vi "Send Core.vi"(6 "Severity Code (info)":T1=enum."info", 8 "Error In":errorcluster, 9 "Message Content":string, 10 "Message Tag":string, 11 "CS++Syslog in":refnum<class "CS++Syslog.lvclass">) -> (0 "Error Out":errorcluster, 3 "CS++Syslog out":refnum<class "CS++Syslog.lvclass">)   [LabVIEW 2014, in "CS++Syslog.lvlib" / "CS++Syslog.lvclass"]
doc: "Send mesage to central message logger."
uses:
  CS++Syslog.lvclass
  CSPP_Core/Libraries/Base/Severity.ctl
  <vilib>/NI/syslog/_subVIs/TypeDefs/syslog_facility_codes.ctl
  CSPP_Core/Libraries/Base/CS++Base.lvlib
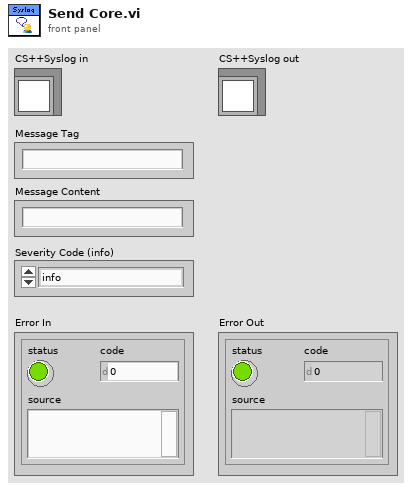
[diagram p1: front panel]
types:
  T1 = typedef "CS++Base.lvlib/Severity.ctl" = enum16{"emergency", "alert", "critical", "error", "warning", "notice", "info", "debug"}
  T2 = typedef "syslog_facility_codes.ctl" = enum16{"kernel", "user", "mail", "system daemons", "security/authorization", "syslogd", "line printer", "network news", "uucp", "clock daemon", "security/authorization (alternate)", "FTP daemon", "NTP subsystem", "log audit", "log alert", "clock daemon (alternate)", "local use 0", "local use 1", "local use 2", "local use 3", "local use 4", "local use 5", "local use 6", "local use 7"}
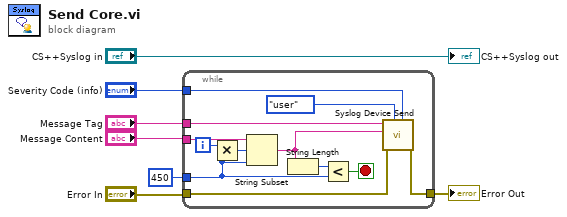
[diagram p0: block diagram]
diagram:
  n1 = while {
    tunnel: "Message Tag" -> [w19]
    tunnel: "Severity Code (info)" -> [w17]
    tunnel: "Error In" -> [w16]
    tunnel: [w15] -> w1
    tunnel: "Message Content" -> [w14]
    tunnel: 450 ("length (rest)") -> [w10]
    i -> [w13]
    stop <- w11 stop-if-true
    n2 = Multiply(x=w13, y=w10) -> (x*y=w12:i32)
    n3 = String Subset(string=w14, offset (0)=w12, length (rest)=w10) -> (substring=w8:string)
    n4 = String Length(string=w8) -> (length=w9:i32)
    n5 = Less?(x=w9, y=w10) -> (x < y?=w11:bool)
    n6 = call <vilib>:"Syslog Device Send.vi"("Severity Code (error)"=w17, "Facility Code (user)"=syslog_facility_codes."user", "error in (no error)"=w16, "Message Content"=w8, "Message Tag"=w19) -> ("error out"=w15:errorcluster)  [unwired: 5 in, 1 out]
  }
  "Error Out" <- w1
  "CS++Syslog out" <- "CS++Syslog in"
